vi "Read Voltage.vi"(8 "Error In":errorcluster, 11 "reference in":refnum<class "PXIe-5172Ref.lvclass">) -> (0 "Error Out":errorcluster, 2 "Voltage":dbl, 3 "reference out":refnum<class "PXIe-5172Ref.lvclass">)   [LabVIEW 2023, in "PXIe-5172.lvlib" / "PXIe-5172Ref.lvclass"]
uses:
  PXIe-5172Ref.lvclass
  PXIe-5172.lvclass
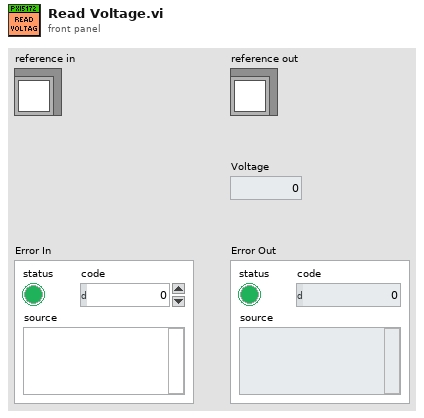
[diagram p1: front panel]
types:
  T1 = typedef "PXIe-5172.lvlib/PXIe-5172Ref.lvclass/ObjectAttributes.ctl" = cluster{"PXIe-5172.lvclass":refnum<class "PXIe-5172.lvclass">}
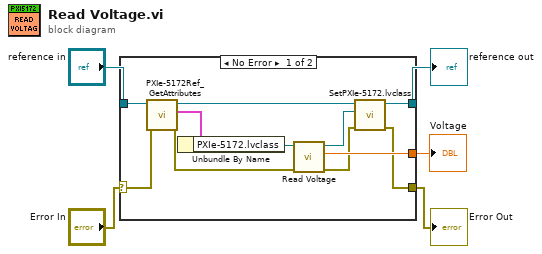
[diagram p0: block diagram]
diagram:
  n1 = case shown="No Error" "Error In" {
    selector: "Error In" -> [w16 w18]
    tunnel: [w7 w18] -> w4
    tunnel: [w9 w17] -> w2
    tunnel: "reference in" -> [w14 w17]
    tunnel: [w11 _] -> w1
    frame No Error {
      n2 = call "PXIe-5172Ref_GetAttributes.vi"("Error In"=w16, "reference in"=w14) -> ("Error Out"=w10:errorcluster, "Data"=w15:T1, "reference out"=w13:refnum<class "PXIe-5172Ref.lvclass">)  [unwired: 6 in, 1 out]
      n3 = Unbundle By Name(w15) -> ("PXIe-5172.lvclass"=w12:refnum<class "PXIe-5172.lvclass">)
      n4 = call-dynamic "Read Voltage.vi"("error in"=w10, "Scope Base in"=w12) -> ("error out"=w8:errorcluster, "Voltage"=w11:dbl, "Scope Base out"=w6:refnum<class "PXIe-5172.lvclass">)  [unwired: 7 in]
      n5 = call "SetPXIe-5172.lvclass.vi"("Error In"=w8, "PXIe-5172.lvclass"=w6, "reference in"=w13) -> ("Error Out"=w7:errorcluster, "reference out"=w9:refnum<class "PXIe-5172Ref.lvclass">)  [unwired: 7 in]
    }
    frame Error {
    }
  }
  "Error Out" <- w4
  "reference out" <- w2
  "Voltage" <- w1
